vi "Main.vi"() -> ()   [LabVIEW 2019]
uses:
  Documents/Demos/ELVIS III/Automated Measurements Board Demo/Common/Dependecies/Function Generator.ctl
  <vilib>/measure/NI_MABase.lvlib
panel:
  in  "?":bool
  out "Signal":waveform(dbl)(graph)
  in  "Signal Generator":T1={"Waveform"=enum."Sine", "DC Offset (V)"=0.0, "Amplitude (V)"=2.0000000000000004, "Frequency (Hz)"=100.0} {"Frequency (Hz)" min=0.0 max=1000.0 step=50.0 format="%#_3p"; "Amplitude (V)" min=0.0 max=5.0 step=0.1; "DC Offset (V)" min=0.0 max=5.0 step=0.1}
  out "?":bool
  in  "?":bool
  # "Remote Front Panel Test"
  # "This VI has the function to demonstrate that a NI RT Target Front Panel can be used remotely."
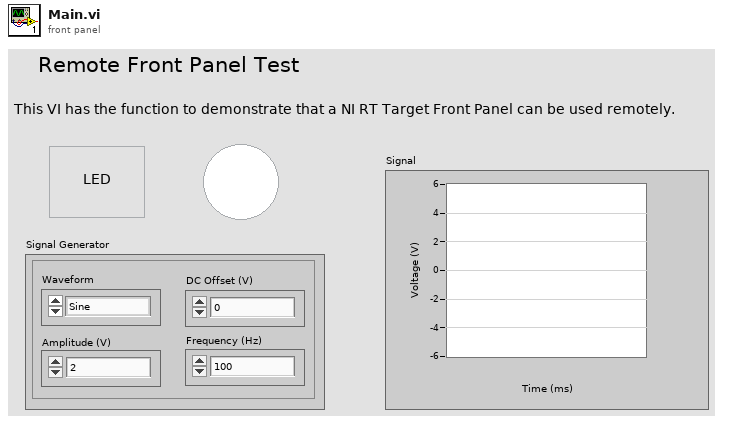
[diagram p1: front panel]
types:
  T1 = typedef "Function Generator.ctl" = cluster{"Waveform":enum16{"Sine", "Square", "Triangle", "DC"}, "DC Offset (V)":dbl, "Amplitude (V)":dbl, "Frequency (Hz)":dbl}
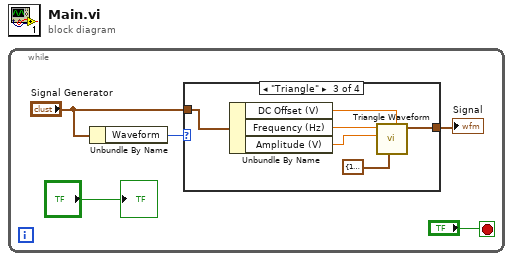
[diagram p0: block diagram]
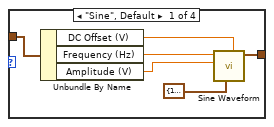
[diagram p2: hidden frame]
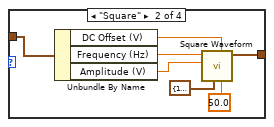
[diagram p3: hidden frame]
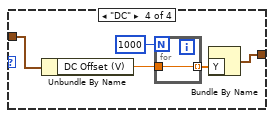
[diagram p4: hidden frame]
diagram:
  n1 = while {
    stop <- "?" stop-if-true
    n2 = Unbundle By Name("Signal Generator") -> ("Waveform"=w4:enum16{"Sine", "Square", "Triangle", "DC"})
    n3 = case shown="\"Triangle\"" w4 {
      tunnel: [w11 w18 w24 w29] -> w5
      tunnel: "Signal Generator" -> [w7 w14 w20 w27]
      frame "Sine", Default {
        n4 = Unbundle By Name(w7) -> ("DC Offset (V)"=w10:dbl, "Frequency (Hz)"=w9:dbl, "Amplitude (V)"=w8:dbl)
        n5 = call <vilib>:"Sine Waveform.vi"("offset"=w10, "sampling info"=cluster{"Fs":dbl, "#s":dbl} {"Fs"=10000.0, "#s"=1000.0}, "amplitude"=w8, "frequency"=w9) -> ("signal out"=w11:waveform(dbl))  [unwired: 6 in, 1 out]
      }
      frame "Square" {
        n6 = Unbundle By Name(w14) -> ("DC Offset (V)"=w17:dbl, "Frequency (Hz)"=w16:dbl, "Amplitude (V)"=w15:dbl)
        n7 = call <vilib>:"Square Waveform.vi"("duty cycle (%)"=50.0, "offset"=w17, "sampling info"=cluster{"Fs":dbl, "#s":dbl} {"Fs"=10000.0, "#s"=1000.0}, "amplitude"=w15, "frequency"=w16) -> ("signal out"=w18:waveform(dbl))  [unwired: 5 in, 1 out]
      }
      frame "Triangle" {
        n8 = Unbundle By Name(w20) -> ("DC Offset (V)"=w23:dbl, "Frequency (Hz)"=w22:dbl, "Amplitude (V)"=w21:dbl)
        n9 = call <vilib>:"Triangle Waveform.vi"("offset"=w23, "sampling info"=cluster{"Fs":dbl, "#s":dbl} {"Fs"=10000.0, "#s"=1000.0}, "amplitude"=w21, "frequency"=w22) -> ("signal out"=w24:waveform(dbl))  [unwired: 6 in, 1 out]
      }
      frame "DC" {
        n10 = Unbundle By Name(w27) -> ("DC Offset (V)"=w26:dbl)
        n11 = for {
          N: 1000 -> [_]
          tunnel: w26 -> [w30]
          tunnel: [w30] -> w28 mode=indexing
        }
        n12 = Bundle By Name("Y"=w28) -> (w29:waveform(dbl))  [unwired: 1 in]
      }
    }
    "Signal" <- w5
    "?" <- "?"
  }
